vi "Parameter Matrix Handler.vi"(5 "Operation (Initialization)":T3, 6 "menu tag":string, 7 "matrix reference":refnum<vi>, 8 "error in (no error)":errorcluster, 9 "Mouse Point":T2, 10 "menu reference":refnum<k9>, 11 "parameters":T1[](array[typedef])) -> (0 "error out":errorcluster, 1 "description":string, 2 "selected tag":string, 3 "parameters out":T1[](array[typedef]))   [LabVIEW 2020]
uses:
  Corr Parameter Item.ctl
  Parameter Matrix Operation.vi
  <vilib>/Utility/miscctls.llb/LVPositionTypeDef.ctl
  <vilib>/Utility/miscctls.llb/LVRowAndColumnTypeDef.ctl
  <vilib>/Utility/miscctls.llb/LVBoundsTypeDef.ctl
panel:
  in  "default all label":string="<default all>"
  in  "default label":string="<default>"
  in  "clear all label":string="<clear all>"
  in  "clear label":string="<clear>"
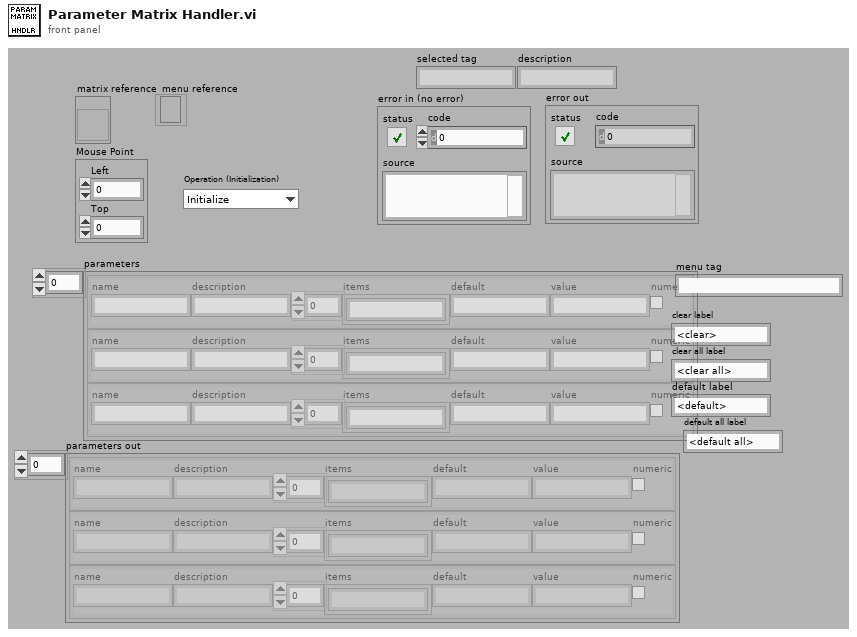
[diagram p1: front panel]
types:
  T1 = typedef "Corr Parameter Item.ctl" = cluster{"name":string, "description":string, "items":string[], "default":string, "value":string, "numeric":bool}
  T2 = typedef "LVPositionTypeDef.ctl" = cluster{"Left":i32, "Top":i32}
  T3 = typedef "Parameter Matrix Operation.vi" = enum16{"Initialize", "On Row Select", "On Menu Drop", "On Menu Select", "Get values"}
  T4 = typedef "LVRowAndColumnTypeDef.ctl" = cluster{"Row":i32, "Column":i32}
  T5 = typedef "LVBoundsTypeDef.ctl" = cluster{"Width":u32, "Height":u32}
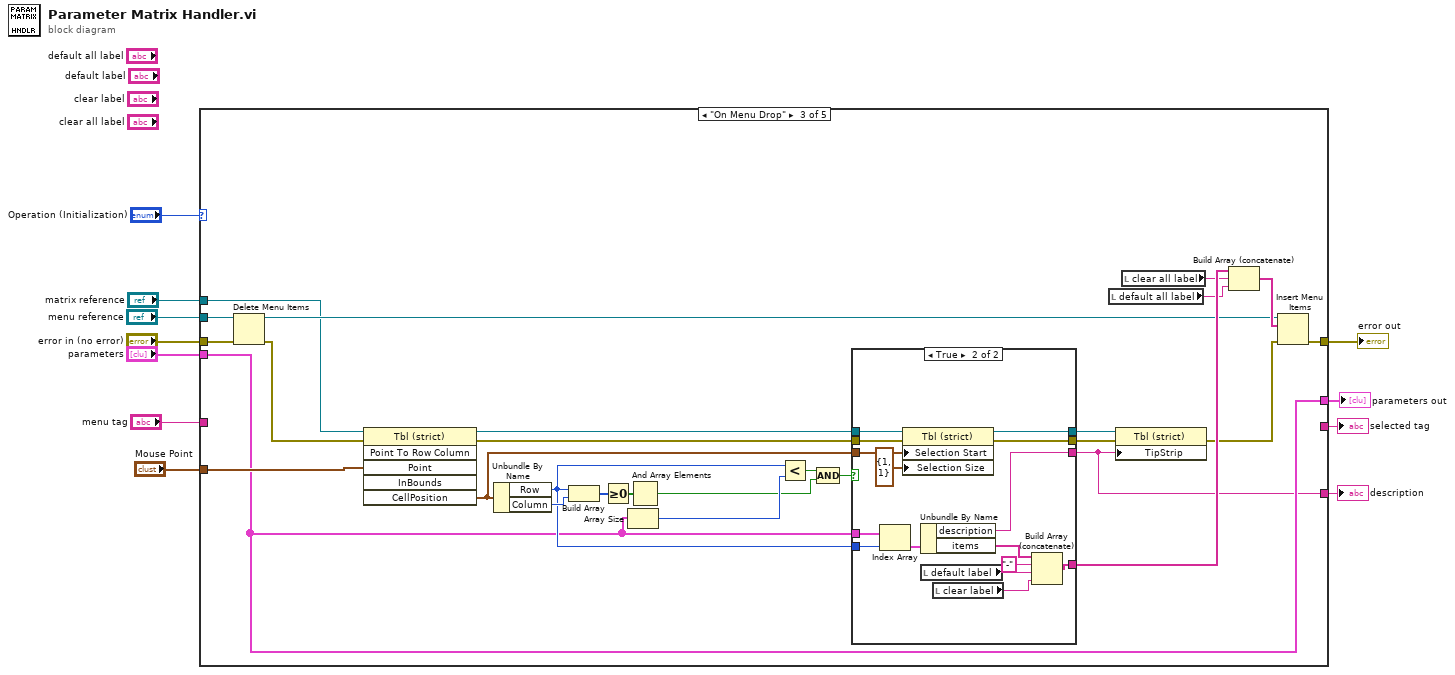
[diagram p0: block diagram]
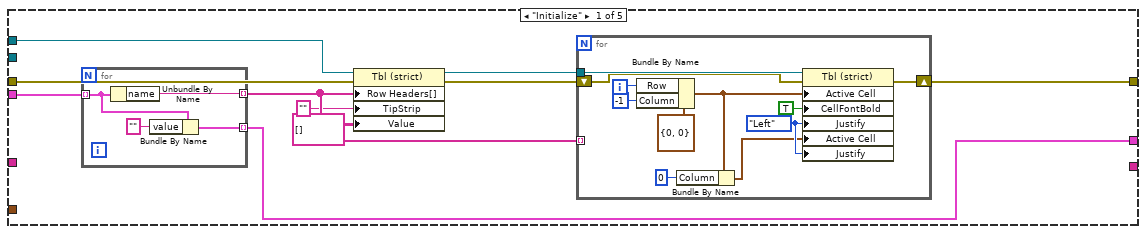
[diagram p2: hidden frame]
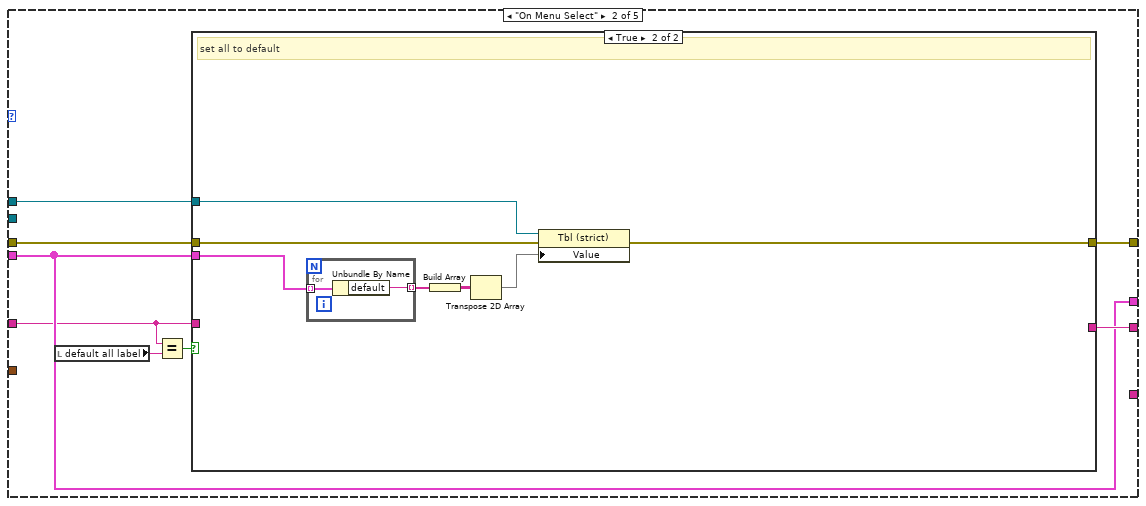
[diagram p3: hidden frame]
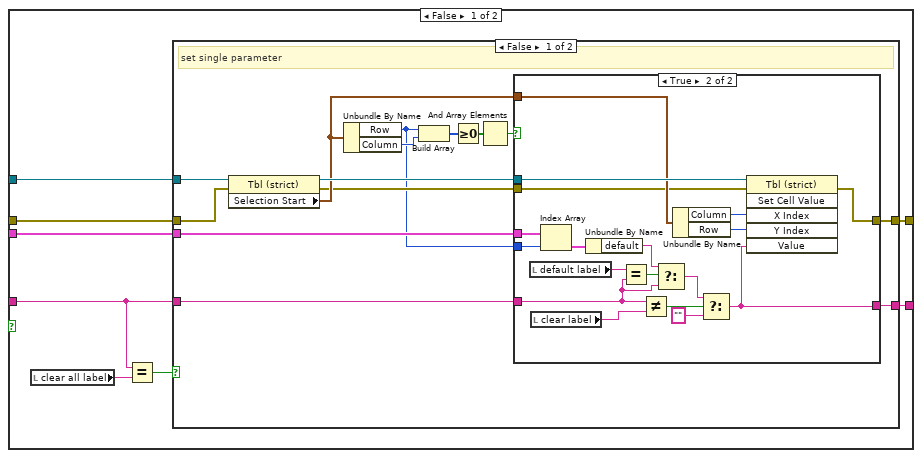
[diagram p4: hidden frame]
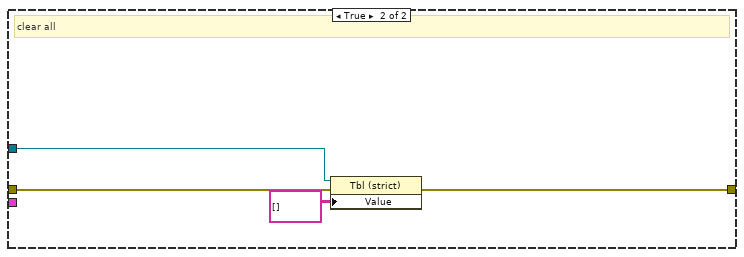
[diagram p6: hidden frame]
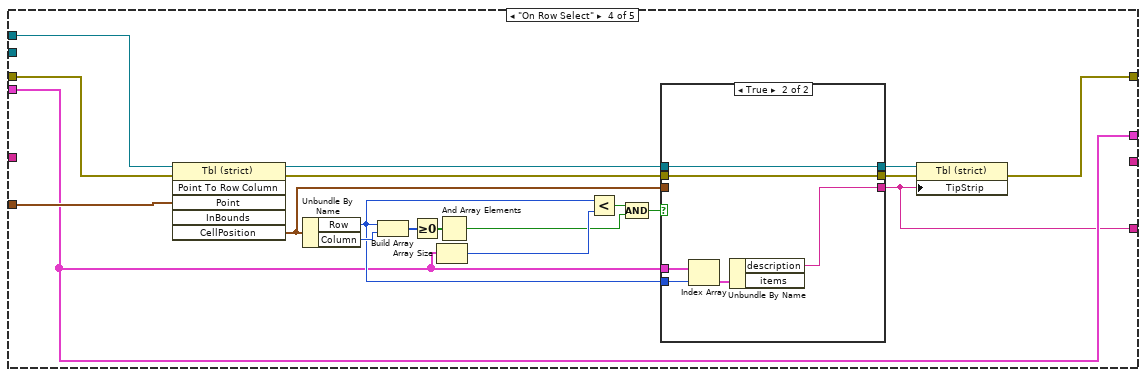
[diagram p8: hidden frame]
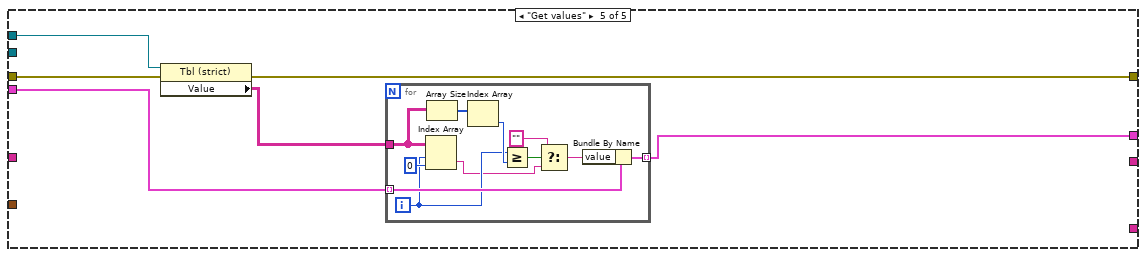
[diagram p10: hidden frame]
diagram:
  n1 = case shown="\"On Menu Drop\"" "Operation (Initialization)" {
    tunnel: "parameters" -> [w13 w40 w101 w144 w170]
    tunnel: "matrix reference" -> [w18 w44 w117 w156 w174]
    tunnel: "error in (no error)" -> [w16 w43 w114 w146 w175]
    tunnel: [w15 w42 w111 w145 w173] -> w7
    tunnel: "menu reference" -> [_ _ w116 _ _]
    tunnel: "Mouse Point" -> [_ _ w113 w155 _]
    tunnel: "menu tag" -> [_ w38 _ _ _]
    tunnel: [_ w41 _ _ _] -> w3
    tunnel: [w12 w40 w101 w144 w171] -> w2
    tunnel: [_ _ w100 w143 _] -> w1
    frame "Initialize" {
      n2 = for {
        tunnel: w13 -> [w35] mode=indexing
        tunnel: [w36] -> w20 mode=indexing
        tunnel: [w33] -> w12 mode=indexing
        n3 = Unbundle By Name(w35) -> ("name"=w36:string)
        n4 = Bundle By Name(cluster=w35, "value"="") -> (w33:T1)
      }
      n5 = property class="Tbl (strict)"(reference=w18, error in=w16, "Row Headers[]"=w20, "TipStrip"="" ("Tip Strip"), "Value"=string[][] []) -> (reference out=w21:refnum<vi>, error out=w17:errorcluster)
      n6 = for {
        tunnel: w20 -> [_] mode=indexing
        tunnel: w21 -> [w32]
        shift-right: [w26] -> w15
        shift-left: w17 -> [w27]
        i -> [w30]
        w25 = enum16{"Left", "Center", "Right"}."Left" ("Active Cell:Cell Justification")
        n7 = Bundle By Name(cluster=T4 {"Row"=0, "Column"=0} ("Active Cell:Active Cell"), "Row"=w30, "Column"=-1) -> (w24:T4)
        n8 = Bundle By Name(cluster=w24, "Column"=0) -> (w23:T4)
        n9 = property class="Tbl (strict)"(reference=w32, error in=w27, "Active Cell"=w24, "CellFontBold"=TRUE ("Active Cell:Cell Font:Bold"), "Justify"=w25, "Active Cell"=w23, "Justify"=w25) -> (error out=w26:errorcluster)  [unwired: 1 out]
      }
    }
    frame "On Menu Select" {
      n10 = local read "default all label"() -> (w39:string)
      n11 = Equal?(x=w38, y=w39) -> (x = y?=w37:bool)
      n12 = case shown="True" w37 {
        tunnel: w44 -> [w52 w94]
        tunnel: w43 -> [w51 w96]
        tunnel: [w50 w95] -> w42
        tunnel: [w49 _] -> w41
        tunnel: w38 -> [w47 _]
        tunnel: w40 -> [w45 w93]
        frame False {
          n13 = local read "clear all label"() -> (w48:string)
          n14 = Equal?(x=w47, y=w48) -> (x = y?=w46:bool)
          n15 = case shown="False" w46 {
            tunnel: w52 -> [w66 w88]
            tunnel: w51 -> [w65 w89]
            tunnel: [w57 w87] -> w50
            tunnel: [w56 _] -> w49
            tunnel: w47 -> [w55 _]
            tunnel: w45 -> [w54 _]
            frame False {
              # "set single parameter"
              n16 = property class="Tbl (strict)"(reference=w66, error in=w65) -> (reference out=w60:refnum<vi>, error out=w58:errorcluster, "Selection Start"=w59:T4)
              n17 = Unbundle By Name(w59) -> ("Row"=w53:i32, "Column"=w62:i32)
              n18 = Build Array(w53, w62) -> (w63:i32[])
              n19 = Greater Or Equal To 0?(x=w63) -> (x >= 0?=w64:bool[])
              n20 = And Array Elements(Boolean array=w64) -> (logical AND=w61:bool)
              n21 = case shown="True" w61 {
                tunnel: w55 -> [_ w68]
                tunnel: w60 -> [_ w83]
                tunnel: w59 -> [_ w82]
                tunnel: w58 -> [w67 w79]
                tunnel: [w67 w78] -> w57
                tunnel: [_ w77] -> w56
                tunnel: w54 -> [_ w76]
                tunnel: w53 -> [_ w75]
                frame False {
                }
                frame True {
                  n22 = local read "default label"() -> (w71:string)
                  n23 = local read "clear label"() -> (w72:string)
                  n24 = Index Array(array=w76, index=w75) -> (element=w70:T1)
                  n25 = Unbundle By Name(w70) -> ("default"=w69:string)
                  n26 = Equal?(x=w71, y=w68) -> (x = y?=w73:bool)
                  n27 = Not Equal?(x=w68, y=w72) -> (x != y?=w85:bool)
                  n28 = Select(t=w69, s=w73, f=w68) -> (s? t:f=w74:string)
                  n29 = Unbundle By Name(w82) -> ("Column"=w81:i32, "Row"=w80:i32)
                  n30 = Select(t=w74, s=w85, f="") -> (s? t:f=w77:string)
                  n31 = invoke class="Tbl (strict)" method="Set Cell Value"(reference=w83, error in=w79, "X Index"=w81, "Y Index"=w80, "Value"=w77) -> (error out=w78:errorcluster)  [unwired: 1 in, 5 out]
                }
              }
            }
            frame True {
              # "clear all"
              n32 = property class="Tbl (strict)"(reference=w88, error in=w89, "Value"=string[][] []) -> (error out=w87:errorcluster)  [unwired: 1 out]
            }
          }
        }
        frame True {
          # "set all to default"
          n33 = for {
            tunnel: w93 -> [w98] mode=indexing
            tunnel: [w97] -> w92 mode=indexing
            n34 = Unbundle By Name(w98) -> ("default"=w97:string)
          }
          n35 = Build Array(w92) -> (w91:string[][])
          n36 = Transpose 2D Array(2D array=w91) -> (transposed array=w90:string[][])
          n37 = property class="Tbl (strict)"(reference=w94, error in=w96, "Value"=w90) -> (error out=w95:errorcluster)  [unwired: 1 out]
        }
      }
    }
    frame "On Menu Drop" {
      n38 = Delete Menu Items(6:w114, 9:w116) -> (0:w115:errorcluster, 3:w118:refnum<k9>)  [unwired: 2 in]
      n39 = invoke class="Tbl (strict)" method="Point To Row Column"(reference=w117, error in=w115, "Point"=w113) -> (reference out=w122:refnum<vi>, error out=w112:errorcluster, "CellPosition"=w123:T4)  [unwired: 3 in, 3 out]
      n40 = Unbundle By Name(w123) -> ("Row"=w110:i32, "Column"=w119:i32)
      n41 = Build Array(w110, w119) -> (w120:i32[])
      n42 = Greater Or Equal To 0?(x=w120) -> (x >= 0?=w121:bool[])
      n43 = Array Size(array=w101) -> (size(s)=w109:i32)
      n44 = And Array Elements(Boolean array=w121) -> (logical AND=w107:bool)
      n45 = Less?(x=w110, y=w109) -> (x < y?=w108:bool)
      n46 = Compound Arithmetic op=AND(w108, w107) -> (w106:bool)
      n47 = case shown="True" w106 {
        tunnel: w122 -> [w126 w142]
        tunnel: w123 -> [_ w141]
        tunnel: w101 -> [_ w139]
        tunnel: w110 -> [_ w138]
        tunnel: [_ w131] -> w124
        tunnel: w112 -> [w127 w136]
        tunnel: [w127 w135] -> w105
        tunnel: [w126 w134] -> w104
        tunnel: [_ w133] -> w100
        frame False {
        }
        frame True {
          n48 = Index Array(array=w139, index=w138) -> (element=w137:T1)
          n49 = property class="Tbl (strict)"(reference=w142, error in=w136, "Selection Start"=w141, "Selection Size"=T5 {"Width"=1, "Height"=1} ("Size")) -> (reference out=w134:refnum<vi>, error out=w135:errorcluster)
          n50 = Unbundle By Name(w137) -> ("description"=w133:string, "items"=w132:string[])
          n51 = local read "default label"() -> (w130:string)
          n52 = local read "clear label"() -> (w129:string)
          n53 = Build Array (concatenate)(w132, "-", w130, w129) -> (w131:string[])
        }
      }
      n54 = local read "default all label"() -> (w99:string)
      n55 = property class="Tbl (strict)"(reference=w104, error in=w105, "TipStrip"=w100) -> (error out=w102:errorcluster)  [unwired: 1 out]
      n56 = local read "clear all label"() -> (w103:string)
      n57 = Build Array (concatenate)(w124, w103, w99) -> (w125:string[])
      n58 = Insert Menu Items(6:w102, 8:w125, 9:w118) -> (0:w111:errorcluster)  [unwired: 3 in, 2 out]
    }
    frame "On Row Select" {
      n59 = invoke class="Tbl (strict)" method="Point To Row Column"(reference=w156, error in=w146, "Point"=w155) -> (reference out=w160:refnum<vi>, error out=w154:errorcluster, "CellPosition"=w161:T4)  [unwired: 3 in, 3 out]
      n60 = Unbundle By Name(w161) -> ("Row"=w153:i32, "Column"=w157:i32)
      n61 = Build Array(w153, w157) -> (w158:i32[])
      n62 = Greater Or Equal To 0?(x=w158) -> (x >= 0?=w159:bool[])
      n63 = Array Size(array=w144) -> (size(s)=w152:i32)
      n64 = And Array Elements(Boolean array=w159) -> (logical AND=w150:bool)
      n65 = Less?(x=w153, y=w152) -> (x < y?=w151:bool)
      n66 = Compound Arithmetic op=AND(w151, w150) -> (w149:bool)
      n67 = case shown="True" w149 {
        tunnel: w160 -> [w162 w164]
        tunnel: w161 -> [_ _]
        tunnel: w144 -> [_ w169]
        tunnel: w153 -> [_ w168]
        tunnel: w154 -> [w163 w165]
        tunnel: [w163 w165] -> w148
        tunnel: [w162 w164] -> w147
        tunnel: [_ w166] -> w143
        frame False {
        }
        frame True {
          n68 = Index Array(array=w169, index=w168) -> (element=w167:T1)
          n69 = Unbundle By Name(w167) -> ("description"=w166:string)  [unwired: 1 out]
        }
      }
      n70 = property class="Tbl (strict)"(reference=w147, error in=w148, "TipStrip"=w143) -> (error out=w145:errorcluster)  [unwired: 1 out]
    }
    frame "Get values" {
      n71 = property class="Tbl (strict)"(reference=w174, error in=w175) -> (error out=w173:errorcluster, "Value"=w172:string[][])  [unwired: 1 out]
      n72 = for {
        tunnel: w172 -> [w183]
        tunnel: w170 -> [w186] mode=indexing
        tunnel: [w185] -> w171 mode=indexing
        i -> [w180]
        n73 = Index Array(array=w183, index (row)=w180, index (col)=0 ("disabled index (col)")) -> (element=w178:string)
        n74 = Array Size(array=w183) -> (size(s)=w182:i32[])
        n75 = Index Array(array=w182) -> (element=w181:i32)  [unwired: 1 in]
        n76 = Greater Or Equal?(x=w180, y=w181) -> (x >= y?=w179:bool)
        n77 = Select(t="", s=w179, f=w178) -> (s? t:f=w177:string)
        n78 = Bundle By Name(cluster=w186, "value"=w177) -> (w185:T1)
      }
    }
  }
  "error out" <- w7
  "selected tag" <- w3
  "parameters out" <- w2
  "description" <- w1
